vi "DSF.Engine.Framework.Create.Transfers.vi"(5 "Group String Buffer":refnum<class "DSF.Engine.Memory.Buffer.lvclass">, 7 "Group Engine Buffer":refnum<class "DSF.Engine.Pointer.DBL.lvclass">, 8 "error in (no error)":errorcluster, 10 "Transfer Configurations":refnum<class "DSF.Shared.Configuration.Transfer.lvclass">[](array[class]), 11 "Framework in":refnum<class "DSF.Engine.Framework.lvclass">) -> (0 "error out":errorcluster, 2 "Transfers":refnum<class "DSF.Engine.Transfer.lvclass">[](array[class]), 3 "Framework out":refnum<class "DSF.Engine.Framework.lvclass">)   [LabVIEW 2017, in "DSF.Engine.lvlib" / "DSF.Engine.Framework.lvclass"]
uses:
  DSF.Engine.Framework.lvclass
  Transfer/DSF.Engine.Transfer.lvclass
  Shared/Classes/Transfer/DSF.Shared.Configuration.Transfer.lvclass
  Buffer/DSF.Engine.Memory.Buffer.lvclass
  Pointer/DSF.Engine.Pointer.DBL.lvclass
  C:/Git/DSF/DSF Core/Built/Core/Memory Manager.lvlibp/1abvi3w/vi.lib/National Instruments/Memory Manager/Classes/Pointer/Memory.Pointer.lvclass
  DSF.Engine.Framework.lvclass/DSF.Engine.Framework.ctl
  Cache/DSF.Engine.Memory.Cache.lvclass/DSF.Engine.Memory.Cache.ctl
  DSF Configuration API/1.0.0/Public/Controls/DSF Data Type.ctl
  Shared/Classes/Transfer/DSF.Shared.Configuration.Transfer.lvclass/DSF.Shared.Configuration.Transfer.ctl
  Shared/VIs/DSF.Shared.Data Type.Sizeof.vi
  Built/Core/Memory Manager.lvlibp/1abvi3w/vi.lib/National Instruments/Memory Manager/Classes/Pointer/Memory.Pointer.New.1B.vi
  Built/Core/Memory Manager.lvlibp/1abvi3w/vi.lib/National Instruments/Memory Manager/Classes/Pointer/Memory.Pointer.lvclass
  Cache/DSF.Engine.Memory.Cache.lvclass
  DSF Configuration API/1.0.0/DSF Configuration API.lvlib
  DSF.Engine.lvlib
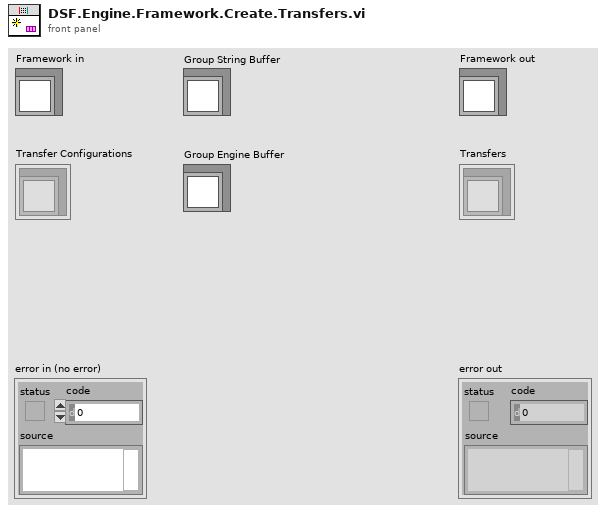
[diagram p1: front panel]
types:
  T1 = typedef "DSF Configuration API.lvlib/DSF Data Type.ctl" = enum8{"Bool", "SGL", "DBL", "I8", "I16", "I32", "I64", "U8", "U16", "U32", "U64"}
  T2 = typedef "DSF.Engine.lvlib/DSF Runtime Channel Block.ctl" = cluster{"data type":T1, "count":u64, "buffer offset":u64}
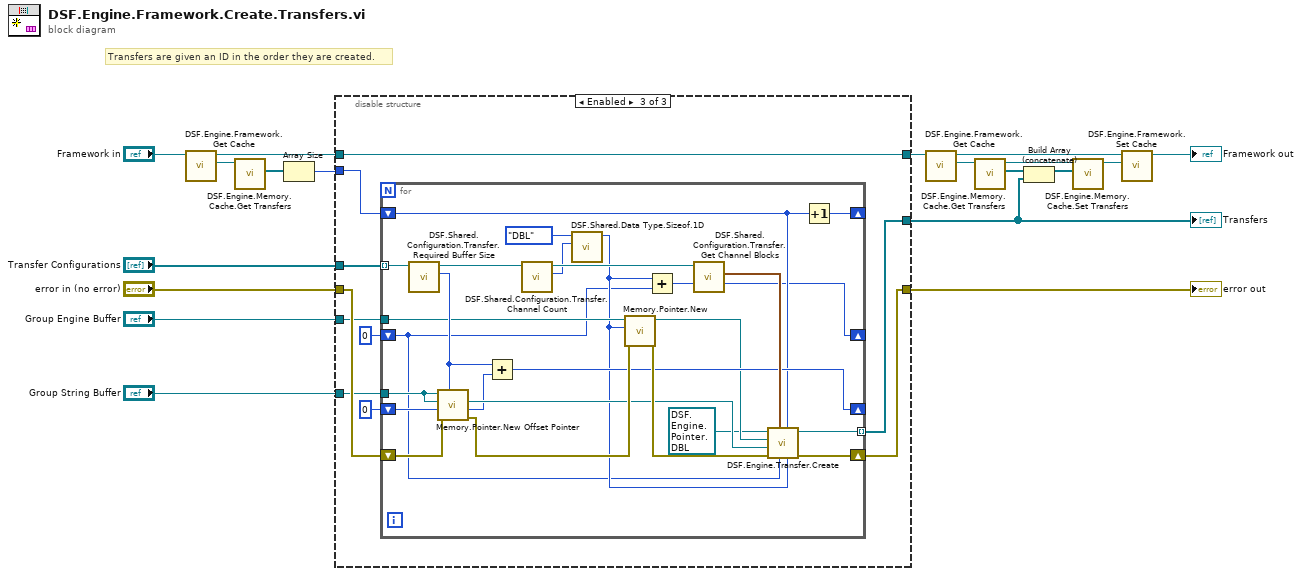
[diagram p0: block diagram]
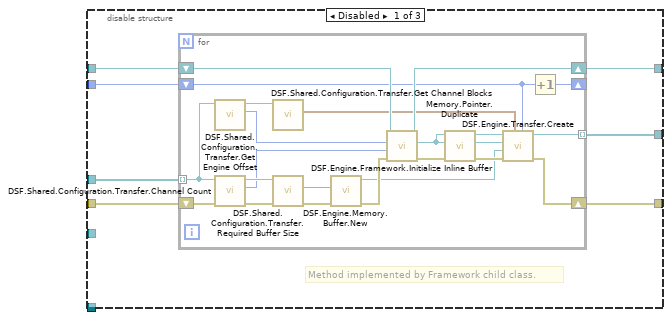
[diagram p2: hidden frame]
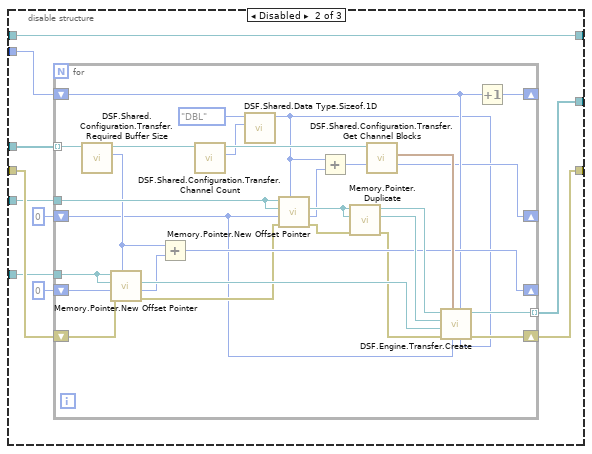
[diagram p3: hidden frame]
diagram:
  # "Transfers are given an ID in the order they are created."
  n1 = call "DSF.Engine.Framework.Get Cache.vi"("Framework in"="Framework in") -> ("Cache"=w12:refnum<class "DSF.Engine.Memory.Cache.lvclass">, "Framework out"=w13:refnum<class "DSF.Engine.Framework.lvclass">)  [unwired: 9 in]
  n2 = call "DSF.Engine.Memory.Cache.Get Transfers.vi"("Cache in"=w12) -> ("Transfers"=w15:refnum<class "DSF.Engine.Transfer.lvclass">[])  [unwired: 9 in, 1 out]
  n3 = Array Size(array=w15) -> (size(s)=w16:i32)
  n4 = disable-structure shown="Enabled" {
    disable-tunnel: [w26 w55 w93] -> w19
    disable-tunnel: "Transfer Configurations" -> [w25 w59 w97]
    disable-tunnel: "error in (no error)" -> [w24 w54 w92]
    disable-tunnel: w16 -> [w23 w57 w95]
    disable-tunnel: w13 -> [w22 w58 w96]
    disable-tunnel: [w21 w58 w96] -> w10
    disable-tunnel: [w20 w56 w94] -> w8
    disable-tunnel: "Group String Buffer" -> [_ w53 w91]
    disable-tunnel: "Group Engine Buffer" -> [_ w52 w90]
    frame Disabled {
      # "Method implemented by Framework child class."
      n5 = for {
        shift-right: [w49] -> w26
        shift-left: w24 -> [w32]
        tunnel: [w48] -> w20 mode=indexing
        shift-right: [w37] -> w21
        shift-left: w22 -> [w47]
        tunnel: w25 -> [w45] mode=indexing
        shift-right: [w30] -> _
        shift-left: w23 -> [w29]
        n6 = call "DSF.Shared.Configuration.Transfer.Get Engine Offset.vi"("Transfer Configuration in"=w45) -> ("engine offset"=w46:u64, "Transfer Configuration out"=w28:refnum<class "DSF.Shared.Configuration.Transfer.lvclass">)  [unwired: 9 in]
        n7 = call "DSF.Shared.Configuration.Transfer.Channel Count.vi"("error in (no error)"=w32, "Transfer Configuration in"=w45) -> ("error out"=w33:errorcluster, "total channel count"=w38:u64, "Transfer Configuration out"=w39:refnum<class "DSF.Shared.Configuration.Transfer.lvclass">)  [unwired: 7 in]
        n8 = call "DSF.Shared.Configuration.Transfer.Get Channel Blocks.vi"("Transfer Configuration in"=w28) -> ("channel blocks"=w27:T2[])  [unwired: 9 in, 1 out]
        n9 = call "DSF.Shared.Configuration.Transfer.Required Buffer Size.vi"("error in (no error)"=w33, "Transfer Configuration in"=w39) -> ("error out"=w31:errorcluster, "required buffer size"=w35:u64)  [unwired: 7 in, 1 out]
        n10 = call "DSF.Engine.Memory.Buffer.New.vi"("error in (no error)"=w31, "size"=w35) -> ("error out"=w36:errorcluster, "Buffer out"=w34:refnum<class "DSF.Engine.Memory.Buffer.lvclass">)  [unwired: 8 in]
        n11 = call-dynamic "DSF.Engine.Framework.Initialize Inline Buffer.vi"("error in (no error)"=w36, "channel count"=w38, "first channel offset"=w46, "Framework in"=w47) -> ("error out"=w40:errorcluster, "Buffer"=w41:refnum<class "DSF.Engine.Pointer.DBL.lvclass">, "Framework out"=w37:refnum<class "DSF.Engine.Framework.lvclass">)  [unwired: 5 in]
        n12 = call "Memory.Pointer.Duplicate.vi"("error in (no error)"=w40, "new Pointer type"=w41, "Pointer in"=w41) -> ("error out"=w44:errorcluster, "new duplicate Pointer"=w43:refnum<class "DSF.Engine.Pointer.DBL.lvclass">, "Pointer out"=w42:refnum<class "DSF.Engine.Pointer.DBL.lvclass">)  [unwired: 6 in]
        n13 = call "DSF.Engine.Transfer.Create.vi"("id"=w29, "channel blocks"=w27, "error in (no error)"=w44, "String Buffer"=w34, "Intermediate Buffer"=w43, "Inline Buffer"=w42) -> ("error out"=w49:errorcluster, "Transfer out"=w48:refnum<class "DSF.Engine.Transfer.lvclass">)  [unwired: 4 in]
        n14 = Increment(x=w29) -> (x+1=w30:i32)
      }
    }
    frame Disabled {
      n15 = for {
        shift-right: [w87] -> w55
        shift-left: w54 -> [w72]
        tunnel: [w86] -> w56 mode=indexing
        tunnel: w59 -> [w80] mode=indexing
        tunnel: w52 -> [w85]
        shift-right: [w63] -> _
        shift-left: u64 0 -> [w61]
        tunnel: w53 -> [w70]
        shift-right: [w74] -> _
        shift-left: u64 0 -> [w78]
        shift-right: [w65] -> _
        shift-left: w57 -> [w64]
        n16 = call "DSF.Shared.Configuration.Transfer.Required Buffer Size.vi"("Transfer Configuration in"=w80) -> ("required buffer size"=w77:u64, "Transfer Configuration out"=w79:refnum<class "DSF.Shared.Configuration.Transfer.lvclass">)  [unwired: 8 in, 1 out]
        n17 = call "Memory.Pointer.New Offset Pointer.vi"("length (-1: rest)"=w77, "error in (no error)"=w72, "offset (0)"=w78, "offset Pointer type"=w70, "base Pointer in"=w70) -> ("error out"=w68:errorcluster, "offset out"=w71:u64, "offset Pointer"=w76:refnum<class "DSF.Engine.Memory.Buffer.lvclass">)  [unwired: 3 in, 1 out]
        n18 = Add(x=w77, y=w71) -> (x+y=w74:u64)
        n19 = call "DSF.Shared.Configuration.Transfer.Channel Count.vi"("Transfer Configuration in"=w79) -> ("total channel count"=w69:u64, "Transfer Configuration out"=w73:refnum<class "DSF.Shared.Configuration.Transfer.lvclass">)  [unwired: 8 in, 1 out]
        n20 = call "DSF.Shared.Data Type.Sizeof.1D.vi"("count"=w69, "data type"=DSF_Data_Type."DBL") -> ("size in bytes"=w60:u64)  [unwired: 9 in]
        n21 = call "Memory.Pointer.New Offset Pointer.vi"("length (-1: rest)"=w60, "error in (no error)"=w68, "offset (0)"=w61, "offset Pointer type"=w85, "base Pointer in"=w85) -> ("error out"=w67:errorcluster, "offset out"=w62:u64, "offset Pointer"=w82:refnum<class "DSF.Engine.Pointer.DBL.lvclass">)  [unwired: 3 in, 1 out]
        n22 = Add(x=w60, y=w62) -> (x+y=w63:u64)
        n23 = call "Memory.Pointer.Duplicate.vi"("error in (no error)"=w67, "new Pointer type"=w82, "Pointer in"=w82) -> ("error out"=w66:errorcluster, "new duplicate Pointer"=w81:refnum<class "DSF.Engine.Pointer.DBL.lvclass">, "Pointer out"=w83:refnum<class "DSF.Engine.Pointer.DBL.lvclass">)  [unwired: 6 in]
        n24 = call "DSF.Shared.Configuration.Transfer.Get Channel Blocks.vi"("Transfer Configuration in"=w73) -> ("channel blocks"=w75:T2[])  [unwired: 9 in, 1 out]
        n25 = call "DSF.Engine.Transfer.Create.vi"("size"=w60, "id"=w64, "group offset"=w61, "channel blocks"=w75, "error in (no error)"=w66, "String Buffer"=w76, "Intermediate Buffer"=w81, "Inline Buffer"=w83) -> ("error out"=w87:errorcluster, "Transfer out"=w86:refnum<class "DSF.Engine.Transfer.lvclass">)  [unwired: 2 in]
        n26 = Increment(x=w64) -> (x+1=w65:i32)
      }
    }
    frame Enabled {
      n27 = for {
        shift-right: [w120] -> w93
        shift-left: w92 -> [w109]
        tunnel: [w119] -> w94 mode=indexing
        tunnel: w97 -> [w117] mode=indexing
        tunnel: w90 -> [w102]
        shift-right: [w103] -> _
        shift-left: u64 0 -> [w98]
        tunnel: w91 -> [w107]
        shift-right: [w111] -> _
        shift-left: u64 0 -> [w115]
        shift-right: [w105] -> _
        shift-left: w95 -> [w104]
        n28 = call "DSF.Shared.Configuration.Transfer.Required Buffer Size.vi"("Transfer Configuration in"=w117) -> ("required buffer size"=w114:u64, "Transfer Configuration out"=w116:refnum<class "DSF.Shared.Configuration.Transfer.lvclass">)  [unwired: 8 in, 1 out]
        n29 = call "Memory.Pointer.New Offset Pointer.vi"("length (-1: rest)"=w114, "error in (no error)"=w109, "offset (0)"=w115, "offset Pointer type"=w107, "base Pointer in"=w107) -> ("error out"=w122:errorcluster, "offset out"=w108:u64, "offset Pointer"=w113:refnum<class "DSF.Engine.Memory.Buffer.lvclass">)  [unwired: 3 in, 1 out]
        n30 = Add(x=w114, y=w108) -> (x+y=w111:u64)
        n31 = call "DSF.Shared.Configuration.Transfer.Channel Count.vi"("Transfer Configuration in"=w116) -> ("total channel count"=w106:u64, "Transfer Configuration out"=w110:refnum<class "DSF.Shared.Configuration.Transfer.lvclass">)  [unwired: 8 in, 1 out]
        n32 = call "DSF.Shared.Data Type.Sizeof.1D.vi"("count"=w106, "data type"=DSF_Data_Type."DBL") -> ("size in bytes"=w99:u64)  [unwired: 9 in]
        n33 = call-poly "Memory.Pointer.New.vi"("error in (no error)"=w122, "count (1)"=w99, "Pointer type"=w102) -> ("error out"=w121:errorcluster, "Pointer"=w101:refnum<class "DSF.Engine.Pointer.DBL.lvclass">)  [unwired: 7 in]
        n34 = Add(x=w99, y=w98) -> (x+y=w103:u64)
        n35 = call "DSF.Shared.Configuration.Transfer.Get Channel Blocks.vi"("Transfer Configuration in"=w110) -> ("channel blocks"=w112:T2[])  [unwired: 9 in, 1 out]
        n36 = call "DSF.Engine.Transfer.Create.vi"("size"=w99, "id"=w104, "group offset"=w98, "channel blocks"=w112, "error in (no error)"=w121, "String Buffer"=w113, "Intermediate Buffer"=w101, "Inline Buffer"=refnum<class "DSF.Engine.Pointer.DBL.lvclass"> refnum) -> ("error out"=w120:errorcluster, "Transfer out"=w119:refnum<class "DSF.Engine.Transfer.lvclass">)  [unwired: 2 in]
        n37 = Increment(x=w104) -> (x+1=w105:i32)
      }
    }
  }
  "error out" <- w19
  "Transfers" <- w8
  n38 = call "DSF.Engine.Framework.Get Cache.vi"("Framework in"=w10) -> ("Cache"=w11:refnum<class "DSF.Engine.Memory.Cache.lvclass">, "Framework out"=w7:refnum<class "DSF.Engine.Framework.lvclass">)  [unwired: 9 in]
  n39 = call "DSF.Engine.Memory.Cache.Get Transfers.vi"("Cache in"=w11) -> ("Transfers"=w9:refnum<class "DSF.Engine.Transfer.lvclass">[], "Cache out"=w3:refnum<class "DSF.Engine.Memory.Cache.lvclass">)  [unwired: 9 in]
  n40 = Build Array (concatenate)(w9, w8) -> (w6:refnum<class "DSF.Engine.Transfer.lvclass">[])
  n41 = call "DSF.Engine.Memory.Cache.Set Transfers.vi"("Transfers"=w6, "Cache in"=w3) -> ("Cache out"=w5:refnum<class "DSF.Engine.Memory.Cache.lvclass">)  [unwired: 9 in]
  n42 = call "DSF.Engine.Framework.Set Cache.vi"("Cache"=w5, "Framework in"=w7) -> ("Framework out"=→"Framework out":refnum<class "DSF.Engine.Framework.lvclass">)  [unwired: 9 in]
